vi "Edit Station Config Item.vi"(9 "Key 2":string, 10 "Key":string, 11 "Station Config in":T1) -> (3 "Station Config out":T1)   [LabVIEW 2025, in "Full User Interface.lvlib"]
uses:
  Full User Interface.lvlib
  Station Config.ctl
  Station Info.ctl
  Localization/Section.ctl
  Localization/Localization.lvlib
panel:
  in  "Disable":bool caption="禁用"
  in  "Cancel":bool
  in  "OK":bool
  in  "SeqFilename":path caption="序列路径"
  in  "NumberOfSocket":i32=1 caption="总槽位数" min=1 max=255
  out "Station":i32 caption="站名" min=0 step=1
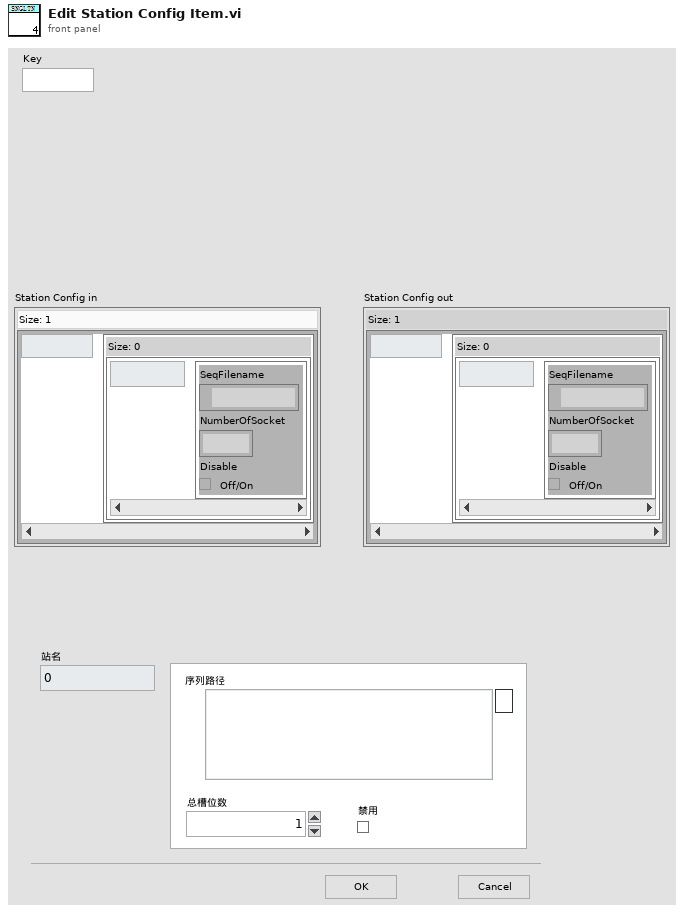
[diagram p1: front panel]
types:
  T1 = typedef "Full User Interface.lvlib/Station Config.ctl" = map{string, map{i32, T2}}
  T2 = typedef "Full User Interface.lvlib/Station Info.ctl" = cluster{"SeqFilename":path, "NumberOfSocket":i32, "Disable":bool}
  T3 = typedef "Localization.lvlib/Section.ctl" = enum16{"Menu", "Title", "Workstation Config"}
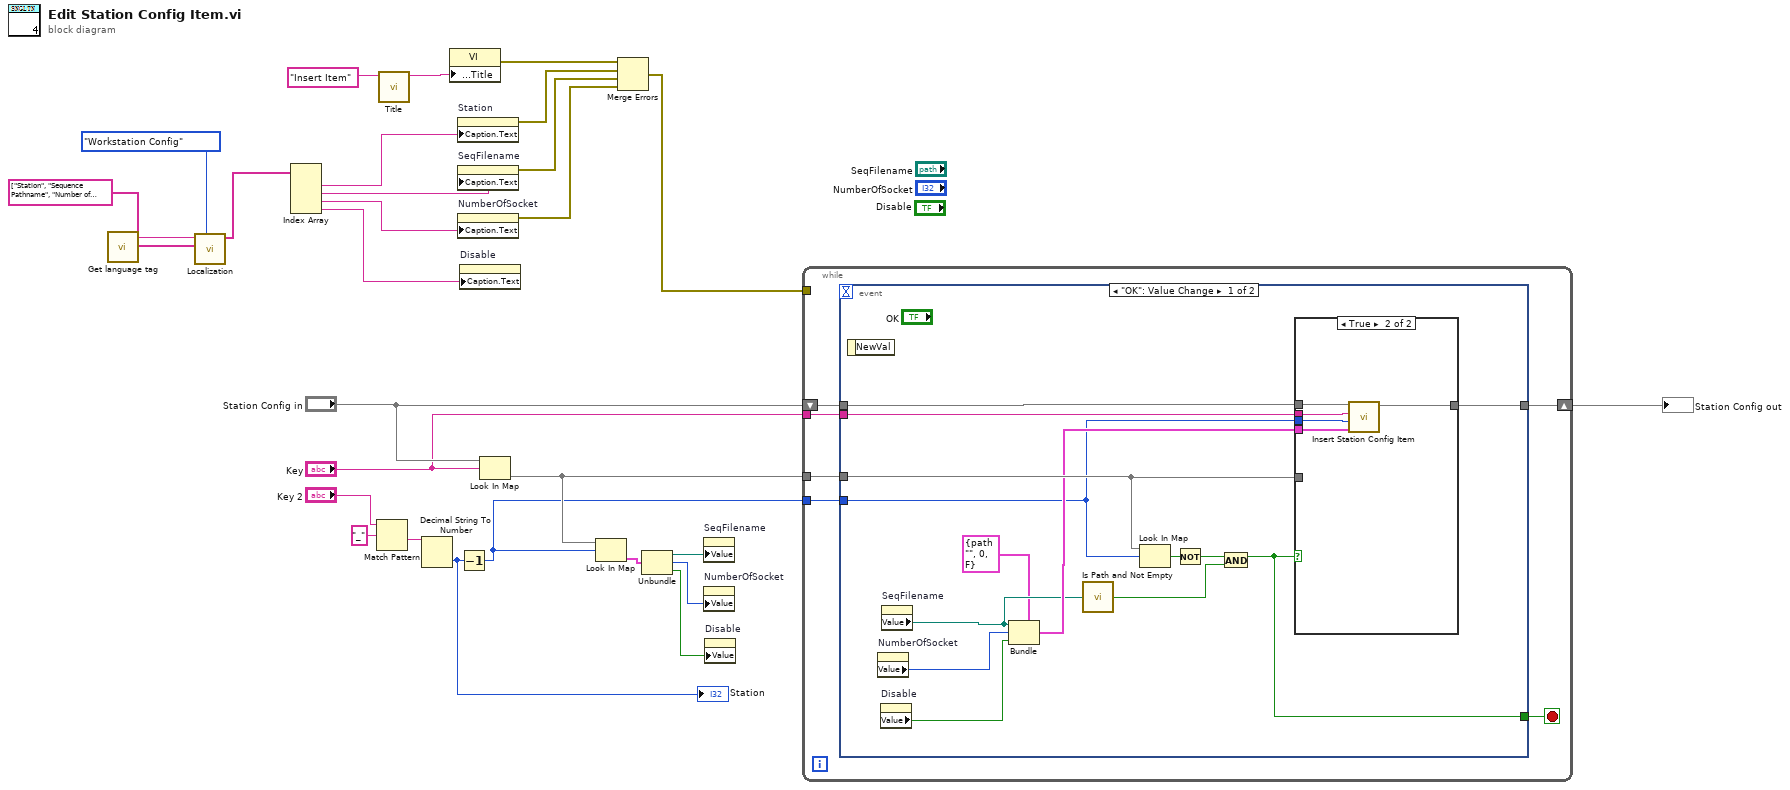
[diagram p0: block diagram]
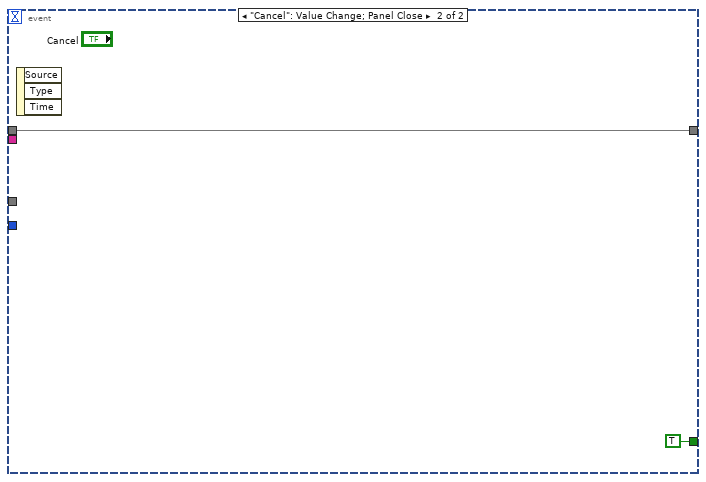
[diagram p3: hidden frame]
diagram:
  n1 = call "Get language tag.vi"() -> ("language tag"=w14:string)  [unwired: 11 in]
  n2 = call "Localization.vi"("section"=Section."Workstation Config", "key"=string[] ["Station", "Sequence Pathname", "Number of Sockets", "Disable"], "Language key"=w14) -> ("Value"=w11:string[])  [unwired: 7 in, 1 out]
  n3 = Index Array(array=w11) -> (element #1=w10:string, element #2=w9:string, element #3=w8:string, element #4=w1:string)  [unwired: 4 in]
  n4 = Match Pattern(string="Key 2", regular expression="_") -> (after substring=w24:string)  [unwired: 1 in, 3 out]
  n5 = call "Title.vi"("Front Panel Window:Title"="Insert Item") -> ("Title"=w15:string)  [unwired: 10 in]
  n6 = Decimal String To Number(string=w24) -> (number=w17:i32)  [unwired: 2 in, 1 out]
  "Station" <- w17
  n7 = property on="Property Node" class="VI"("Front Panel.Title"=w15) -> (error out=w7:errorcluster)  [unwired: 2 in, 1 out]
  n8 = property on="Station" class="DigNum (strict)"("Caption.Text"=w10) -> (error out=w6:errorcluster)  [unwired: 2 in, 1 out]
  n9 = property on="SeqFilename" class="Path"("Caption.Text"=w9) -> (error out=w5:errorcluster)  [unwired: 2 in, 1 out]
  n10 = property on="NumberOfSocket" class="DigNum (strict)"("Caption.Text"=w8) -> (error out=w4:errorcluster)  [unwired: 2 in, 1 out]
  n11 = Decrement(x=w17) -> (x-1=w18:i32)
  n12 = property on="Disable" class="Bool (strict)"("Caption.Text"=w1) -> ()  [unwired: 2 in, 2 out]
  n13 = Look In Map(map="Station Config in", key="Key") -> (value=w23:map{i32, T2})  [unwired: 1 in, 1 out]
  n14 = Look In Map(map=w23, key=w18) -> (value=w22:T2)  [unwired: 1 in, 1 out]
  n15 = Merge Errors(w7, w6, w5, w4) -> (w3:errorcluster)
  n16 = Unbundle(w22) -> ("SeqFilename"=w21:path, "NumberOfSocket"=w20:i32, "Disable"=w2:bool)
  n17 = property on="SeqFilename" class="Path"("Value"=w21) -> ()  [unwired: 2 in, 2 out]
  n18 = property on="NumberOfSocket" class="DigNum (strict)"("Value"=w20) -> ()  [unwired: 2 in, 2 out]
  n19 = property on="Disable" class="Bool (strict)"("Value"=w2) -> ()  [unwired: 2 in, 2 out]
  n20 = while {
    tunnel: w23 -> [w34]
    tunnel: "Key" -> [w31]
    shift-right: [w32] -> w27
    shift-left: "Station Config in" -> [w33]
    tunnel: w18 -> [w29]
    tunnel: w3 -> [_]
    stop <- w30 stop-if-true
    n21 = event shown="[0] \"OK\": Value Change" {
      selector: _ -> [_ _]
      dyn-events: _ -> [_ _]
      timeout: _ -> [_ _]
      tunnel: w34 -> [w48 _]
      tunnel: w33 -> [w47 w56]
      tunnel: [w46 w56] -> w32
      tunnel: w31 -> [w45 _]
      tunnel: [w41 TRUE] -> w30
      tunnel: w29 -> [w39 _]
      event "OK": Value Change {
        n22 = event-data() -> ()  [unwired: 1 in, 1 out]
        n23 = property on="NumberOfSocket" class="DigNum (strict)"() -> ("Value"=w44:i32)  [unwired: 2 in, 2 out]
        n24 = property on="Disable" class="Bool (strict)"() -> ("Value"=w36:bool)  [unwired: 2 in, 2 out]
        n25 = property on="SeqFilename" class="Path"() -> ("Value"=w42:path)  [unwired: 2 in, 2 out]
        n26 = Bundle(cluster=T2 {"SeqFilename"=path "", "NumberOfSocket"=0, "Disable"=FALSE} ("value"), "SeqFilename"=w42, "NumberOfSocket"=w44, "Disable"=w36) -> (w43:T2)
        n27 = call <vilib>:"Is Path and Not Empty.vi"("path"=w42) -> ("Is Path and Not Empty?"=w40:bool)  [unwired: 4 in]
        n28 = Look In Map(map=w48, key=w39) -> (key not found?=w38:bool)  [unwired: 1 in, 1 out]
        n29 = Not(x=w38) -> (.not. x?=w37:bool)
        n30 = And(x=w37, y=w40) -> (x .and. y?=w41:bool)
        n31 = case shown="True" w41 {
          tunnel: w48 -> [_ _]
          tunnel: w47 -> [w49 w54]
          tunnel: [w49 w53] -> w46
          tunnel: w45 -> [_ w52]
          tunnel: w39 -> [_ w51]
          tunnel: w43 -> [_ w50]
          frame False {
          }
          frame True {
            n32 = call "Insert Station Config Item.vi"("value"=w50, "Station"=w51, "Key"=w52, "Station Config in"=w54) -> ("Station Config out"=w53:T1)  [unwired: 7 in]
          }
        }
      }
      event "Cancel": Value Change; Panel Close {
        n33 = event-data() -> ()  [unwired: 1 in, 3 out]
      }
    }
  }
  "Station Config out" <- w27
